vi "Replace Array Subset (Value).vi"(5 "JSON Array":refnum<class "JSON Value.lvclass">, 7 "index":i32, 9 "new element/subarray":refnum<class "JSON Value.lvclass">, 11 "error in":errorcluster) -> (6 "output JSON Array":refnum<class "JSON Value.lvclass">, 15 "error out":errorcluster)   [LabVIEW 2017, in "JSON Value.lvclass"]
doc: "Replaces an element or subarray in an array at the point you specify in index."
uses:
  JSON Value.lvclass
  JSON Value.lvclass/JSON Value.ctl
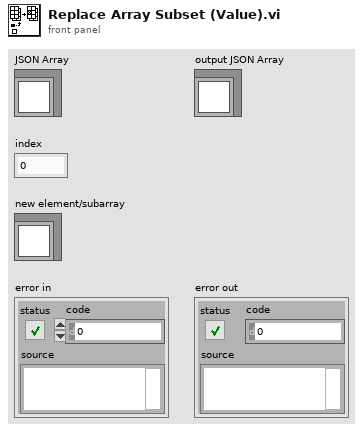
[diagram p1: front panel]
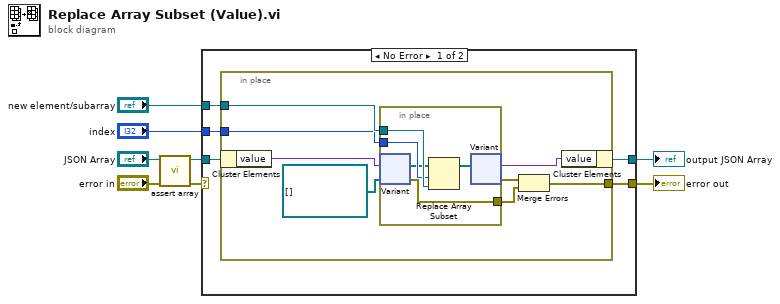
[diagram p0: block diagram]
diagram:
  n1 = call "assert array.vi"("error in (no error)"="error in", "JSON Value in"="JSON Array") -> ("error out"=w3:errorcluster, "JSON Value out"=w1:refnum<class "JSON Value.lvclass">)  [unwired: 8 in]
  n2 = case shown="No Error" w3 {
    selector: w3 -> [_ w28]
    tunnel: w1 -> [w13 w27]
    tunnel: "new element/subarray" -> [w12 _]
    tunnel: "index" -> [w11 _]
    tunnel: [w10 w27] -> w6
    tunnel: [w9 w28] -> w5
    frame No Error {
      n3 = in-place {
        in-place-border: w12 -> [w21]
        in-place-border: w11 -> [w20]
        in-place-border: [w14] -> w9
        n4 = in-place-cluster #1(w13) -> ("value"=w19:variant)
        n5 = in-place {
          in-place-border: w21 -> [w26]
          in-place-border: w20 -> [w25]
          in-place-border: [w22] -> w16
          n6 = in-place-variant #2(w19, refnum<class "JSON Value.lvclass">[] [] ("new element/subarray")) -> (w24:refnum<class "JSON Value.lvclass">[], w22:errorcluster)
          n7 = Replace Array Subset(array=w24, new element=w26, index=w25) -> (w23:refnum<class "JSON Value.lvclass">[])
          n8 = in-place-variant #2(w23) -> (w18:variant, w15:errorcluster)
        }
        n9 = Merge Errors(w15, w16) -> (w14:errorcluster)
        n10 = in-place-cluster #1("value"=w18) -> (w10:refnum<class "JSON Value.lvclass">)
      }
    }
    frame Error {
    }
  }
  "output JSON Array" <- w6
  "error out" <- w5
